vi "Motor_WritePIDGains.vi"(8 "error in (no error)":errorcluster, 10 "PID Gains":T1(array[cluster]), 11 "MotorNew in":refnum<class "MotorControl.lvclass">) -> (0 "error out":errorcluster, 3 "MotorNew out":refnum<class "MotorControl.lvclass">)   [LabVIEW 2014, in "MotorControl.lvclass"]
uses:
  MotorControl.lvclass
  MotorControl.lvclass/MotorControl.ctl
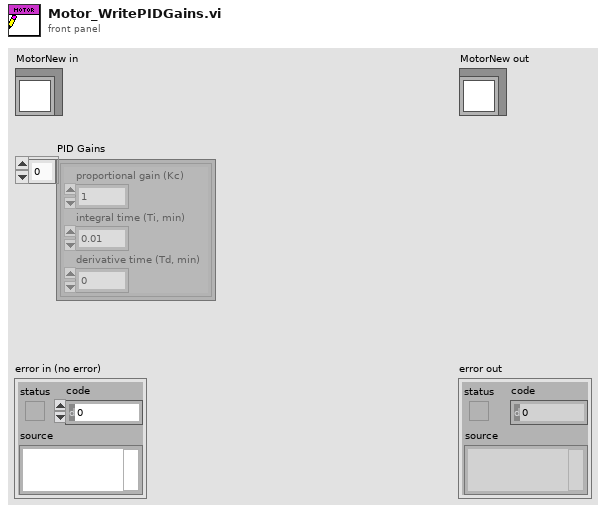
[diagram p1: front panel]
types:
  T1 = cluster{"proportional gain (Kc)":dbl, "integral time (Ti, min)":dbl, "derivative time (Td, min)":dbl}[]
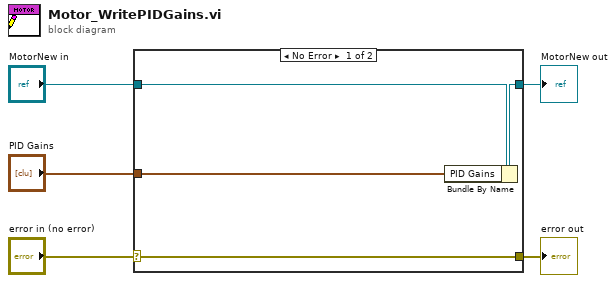
[diagram p0: block diagram]
diagram:
  n1 = case shown="No Error" "error in (no error)" {
    selector: "error in (no error)" -> [w9 w10]
    tunnel: [w9 w10] -> w4
    tunnel: [w7 w11] -> w2
    tunnel: "MotorNew in" -> [w8 w11]
    tunnel: "PID Gains" -> [w6 _]
    frame No Error {
      n2 = Bundle By Name(cluster=w8, "PID Gains"=w6) -> (w7:refnum<class "MotorControl.lvclass">)
    }
    frame Error {
    }
  }
  "error out" <- w4
  "MotorNew out" <- w2
